vi "mcs_main.vi"(10 "MCS Parameters":T1={"Scan Length (Bins)"=64.0, "Dwell Time (s)"=1e-07, "Gate Channel Settings"={"Threshold (V)"=0.0, "Edge"=enum."Falling", "Input Impedence"=enum."1k Ohm"}, "Trig Channel Settings"={"Threshold (V)"=0.0, "Edge"=enum."Falling", "Input Impedence"=enum."1k Ohm"}, "Input 1 Settings"={"Threshold (V)"=0.0, "Edge"=enum."Falling", "Input Impedence"=enum."1k Ohm"}, "Input 2 Settings"={"Threshold (V)"=0.0, "Edge"=enum."Falling", "Input Impedence"=enum."1k Ohm"}, "Number of Sweeps"=1, "Number of Sequential Cycles"=0.0, "Number of Sequences"=0.0, "Sweep Preset"=FALSE, "Sequential Mode"=FALSE, "DAC 1 Ramp Settings"={"Ramp Mode"=enum."Fixed", "Ramp Start Value (V)"=0.0, "Ramp Length (Steps)"=1, "Step Width (bins)"=0, "Step Size (V)"=0.0}, "DAC 2 Output (V)"=0.0, "SYNC Output"=enum."40 MHz Clock", "ROI Min"=0, "ROI Max"=1, "Dual MCS Mode"=FALSE, "DAC 2 Toggle"=FALSE, "MCS on/off"=FALSE, "ROI Max 2"=1, "ROI Min 2"=0, "Sum ROI Only"=FALSE, "Use ROI For \nEach Loop"=FALSE} {"ROI Max 2" min=1; "ROI Min 2" min=0; "ROI Max" min=1; "ROI Min" min=0; "DAC 2 Output (V)" min=-10.0 max=10.0 step=0.00488; "DAC 1 Ramp Settings"."Step Size (V)" min=0.0 max=10.0 step=0.00244 format="%#_4g"; "DAC 1 Ramp Settings"."Step Width (bins)" min=1; "DAC 1 Ramp Settings"."Ramp Length (Steps)" min=1; "DAC 1 Ramp Settings"."Ramp Start Value (V)" min=0.0 max=10.0 step=0.00244; "Number of Sweeps" min=1 step=1 format="%#_6p"; "Input 2 Settings"."Threshold (V)" min=-2.5 max=2.5 step=0.001; "Input 1 Settings"."Threshold (V)" min=-2.5 max=2.5 step=0.001; "Trig Channel Settings"."Threshold (V)" min=-2.5 max=2.5 step=0.001; "Gate Channel Settings"."Threshold (V)" min=-2.5 max=2.5 step=0.001; "Dwell Time (s)" min=1e-07 step=2.5e-08 format="%#_6p"; "Scan Length (Bins)" min=64.0 max=524288.0 format="%#_7f"}) -> ()   [LabVIEW 2015]
uses:
  Controls/MCS/mcs_control_panel.ctl
  Controls/MCS/mcs_channel.ctl
  Controls/MCS/ramp_control.ctl
panel:
  out "array":string[](array[string])
  out "MCS Response":string
  out "MCS Command":string
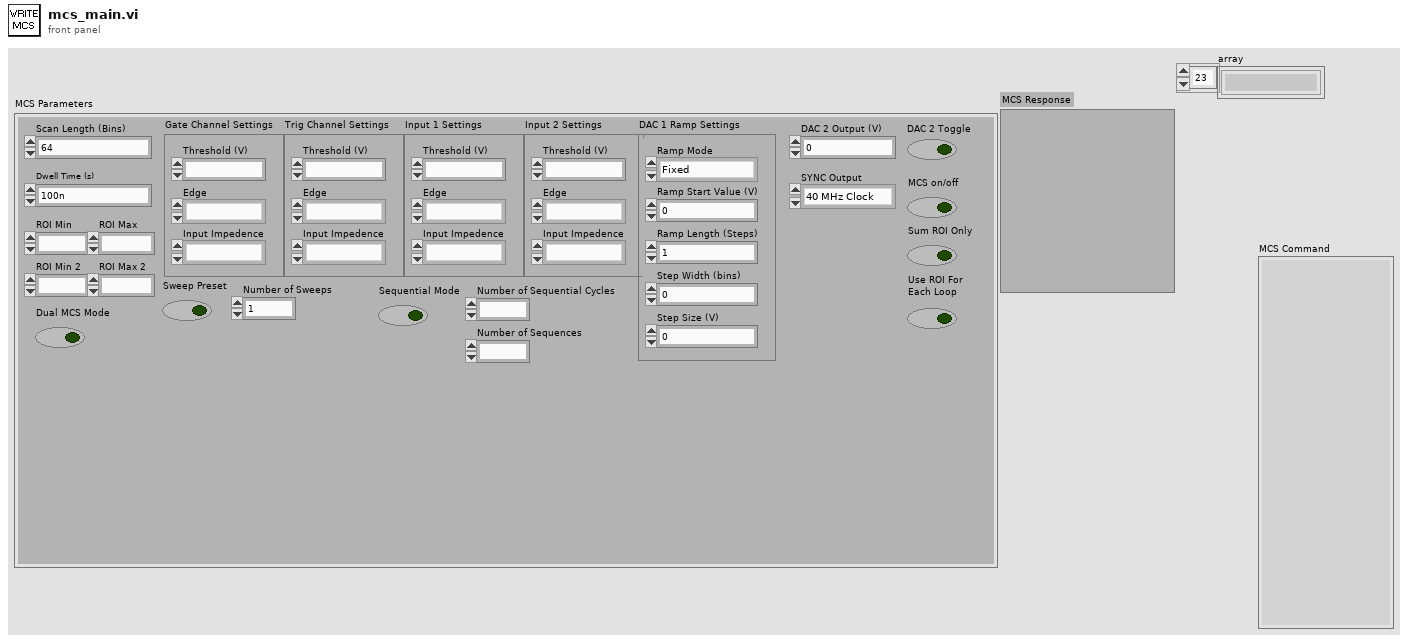
[diagram p1: front panel]
types:
  T1 = typedef "mcs_control_panel.ctl" = cluster{"Scan Length (Bins)":dbl, "Dwell Time (s)":dbl, "Gate Channel Settings":T2, "Trig Channel Settings":T2, "Input 1 Settings":T2, "Input 2 Settings":T2, "Number of Sweeps":i32, "Number of Sequential Cycles":dbl, "Number of Sequences":dbl, "Sweep Preset":bool, "Sequential Mode":bool, "DAC 1 Ramp Settings":T3, "DAC 2 Output (V)":dbl, "SYNC Output":enum16{"40 MHz Clock", "Gate Disc Signal", "Trigger Disc Signal", "Counter 1 Disc Signal", "Counter 2 Disc Signal", "Definitely Not Used", "Not Used", "1 kHz Signal", "Also Not Used", "MCS On/Off", "End of Time Bin", "Ramp Increment Trig", "Step Count Trigger", "'GO'-Line", "Ramp Down Trigger", "Logic 1"}, "ROI Min":i32, "ROI Max":i32, "Dual MCS Mode":bool, "DAC 2 Toggle":bool, "MCS on/off":bool, "ROI Max 2":i32, "ROI Min 2":i32, "Sum ROI Only":bool, "Use ROI For \nEach Loop":bool}
  T2 = typedef "mcs_channel.ctl" = cluster{"Threshold (V)":dbl, "Edge":enum16{"Falling", "Rising"}, "Input Impedence":enum16{"1k Ohm", "50 Ohm"}}
  T3 = typedef "ramp_control.ctl" = cluster{"Ramp Mode":enum16{"Fixed", "Triangle", "Sawtooth"}, "Ramp Start Value (V)":dbl, "Ramp Length (Steps)":i32, "Step Width (bins)":i32, "Step Size (V)":dbl}
  T4 = enum16{"40 MHz Clock", "Gate Disc Signal", "Trigger Disc Signal", "Counter 1 Disc Signal", "Counter 2 Disc Signal", "Definitely Not Used", "Not Used", "1 kHz Signal", "Also Not Used", "MCS On/Off", "End of Time Bin", "Ramp Increment Trig", "Step Count Trigger", "'GO'-Line", "Ramp Down Trigger", "Logic 1"}
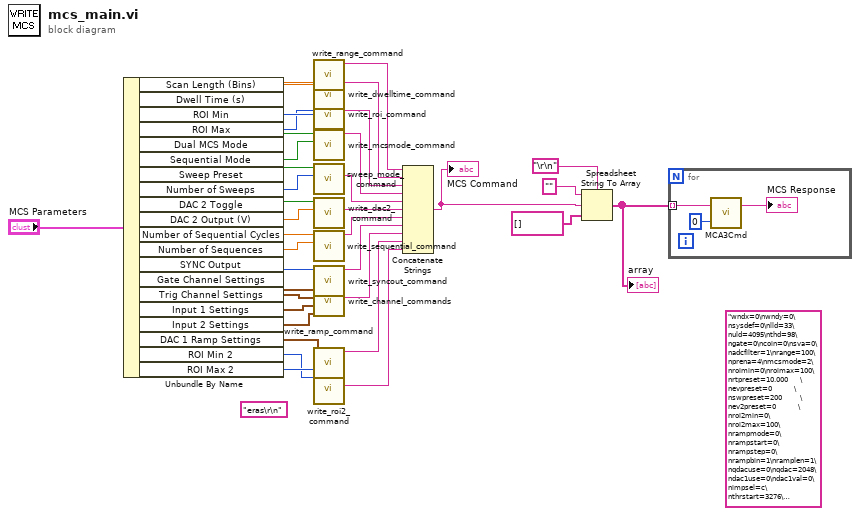
[diagram p0: block diagram]
diagram:
  (unwired) "eras\r\n"
  (unwired) "wndx=0\nwndy=0\nsysdef=0\nlld=33\nuld=4095\nthd=98\ngate=0\ncoin=0\nsva=0\nadcfilter=1\nrange=100\nprena=4\nmcsmode=2\nroimin=0\nroimax=100\nrtpreset=10.000      \nevpreset=0           \nswpreset=200         \nev2preset=0           \nroi2min=0\nroi2max=100\nrampmode=0\nrampstart=0\nrampstep=0\nrampbin=1\nramplen=1\nqdacuse=0\nqdac=2048\ndac1use=0\ndac1val=0\nimpsel=c\nthrstart=3276\nthr1=2457\nthr2=2457\nthrclk=3276\ndiguse=8\ndigval=0\ncycles=0\nsequences=0\nmempart=0\ndwelltime=7\ndwellunit=0\nsyncout=9\nhistlen=0\nautoinc=0 \ndatname=C:\\Users\\Administrator\\Desktop\\UV Data\\Rydberg_to_plasma\\100ms_load_35us_exp_25us_1.asc\nsavedata=0\ndatname2=specB.asc\nsavedata2=0\nfmt=asc\nsmoothpts=5 \ncaluse=0 "
  n1 = Unbundle By Name("MCS Parameters") -> ("Scan Length (Bins)"=w36:dbl, "Dwell Time (s)"=w35:dbl, "ROI Min"=w34:i32, "ROI Max"=w33:i32, "Dual MCS Mode"=w32:bool, "Sequential Mode"=w31:bool, "Sweep Preset"=w30:bool, "Number of Sweeps"=w29:i32, "DAC 2 Toggle"=w28:bool, "DAC 2 Output (V)"=w27:dbl, "Number of Sequential Cycles"=w26:dbl, "Number of Sequences"=w25:dbl, "SYNC Output"=w24:T4, "Gate Channel Settings"=w23:T2, "Trig Channel Settings"=w22:T2, "Input 1 Settings"=w21:T2, "Input 2 Settings"=w20:T2, "DAC 1 Ramp Settings"=w19:T3, "ROI Min 2"=w3:i32, "ROI Max 2"=w4:i32)
  n2 = call "write_range_command.vi"("Scan Length (Bins)"=w36) -> ("Command Out"=w15:string)  [unwired: 10 in]
  n3 = call "write_dwelltime_command.vi"("Dwell Time (s)"=w35) -> ("Command Out"=w16:string)  [unwired: 10 in]
  n4 = call "write_roi_command.vi"("ROI Max"=w33, "ROI Min"=w34) -> ("Command Out"=w17:string)  [unwired: 9 in]
  n5 = call "write_mcsmode_command.vi"("sequential mode"=w31, "dual mcs"=w32) -> ("String"=w9:string)  [unwired: 9 in]
  n6 = call "sweep_mode_command.vi"("Number of Sweeps"=w29, "Sweep Mode"=w30) -> ("Command Out"=w10:string)  [unwired: 9 in]
  n7 = call "write_dac2_command.vi"("dac2 voltage"=w27, "dac2 toggle"=w28) -> ("Command Out"=w18:string)  [unwired: 9 in]
  n8 = call "write_sequential_command.vi"("Number of Sequences"=w25, "Number of Sequential Cycles"=w26) -> ("Command Out"=w14:string)  [unwired: 9 in]
  n9 = call "write_syncout_command.vi"("SYNC Output"=w24) -> ("Command Out"=w13:string)  [unwired: 10 in]
  n10 = call "write_channel_commands.vi"("Input 2 Settings"=w20, "Input 1 Settings"=w21, "Trig Channel Settings"=w22, "Gate Channel Settings"=w23) -> ("Command Out"=w12:string)  [unwired: 7 in]
  n11 = call "write_ramp_command.vi"("DAC 1 Ramp Settings"=w19) -> ("Command Out"=w11:string)  [unwired: 10 in]
  n12 = call "write_roi2_command.vi"("ROI Max"=w4, "ROI Min"=w3) -> ("Command Out"=w2:string)  [unwired: 9 in]
  n13 = Concatenate Strings(w15, w16, w17, w9, w10, w18, w14, w13, w12, w11, w2) -> (w1:string)
  "MCS Command" <- w1
  n14 = Spreadsheet String To Array(delimiter (Tab)="\r\n", format string="", spreadsheet string=w1, array type (2D Dbl)=string[] [] ("Array")) -> (array=w5:string[])
  "array" <- w5
  n15 = for {
    tunnel: w5 -> [w38] mode=indexing
    n16 = call "MCA3Cmd.vi"("MCA #"=0, "Command"=w38) -> ("Response"=→"MCS Response":string)  [unwired: 1 in]
  }
